vi "finishup.vi"(8 "error in (no error)":errorcluster, 11 "PixelflySettings in":refnum<class "PixelflySettings.lvclass">) -> (0 "error out":errorcluster, 3 "PixelflySettings out":refnum<class "PixelflySettings.lvclass">)   [LabVIEW 2011, in "Tools.lvlib" / "Settings.lvlib" / "PixelflySettings.lvclass"]
uses:
  PixelflySettings.lvclass
  PixelflySettings.lvclass/PixelflySettings.ctl
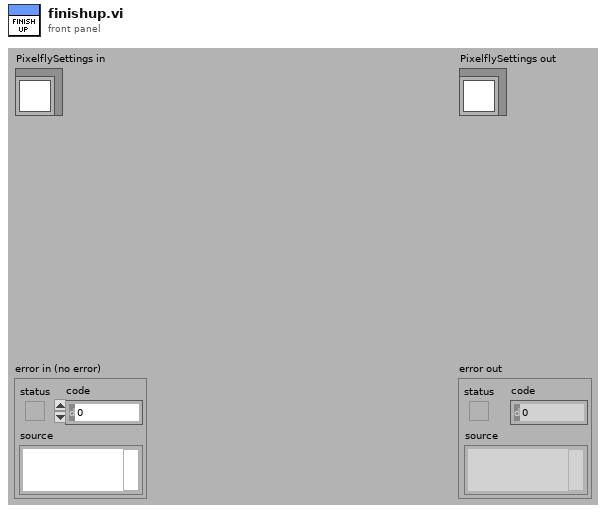
[diagram p1: front panel]
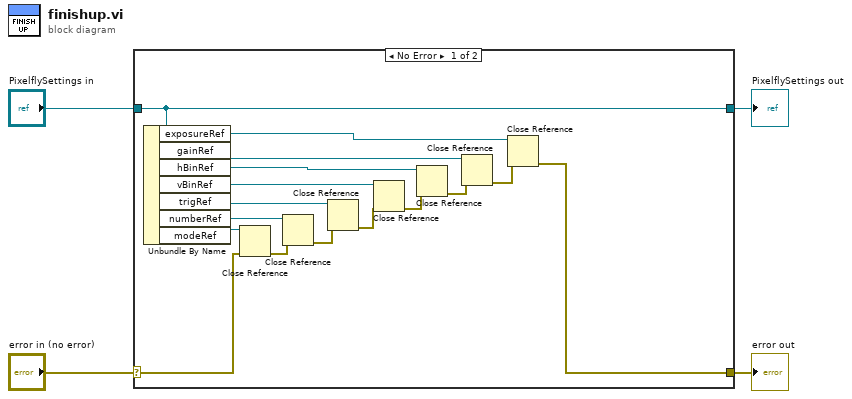
[diagram p0: block diagram]
diagram:
  n1 = case shown="No Error" "error in (no error)" {
    selector: "error in (no error)" -> [w6 w22]
    tunnel: [w5 w22] -> w3
    tunnel: [w20 w21] -> w1
    tunnel: "PixelflySettings in" -> [w20 w21]
    frame No Error {
      n2 = Unbundle By Name(w20) -> ("exposureRef"=w13:refnum<vi>, "gainRef"=w14:refnum<vi>, "hBinRef"=w15:refnum<vi>, "vBinRef"=w16:refnum<vi>, "trigRef"=w17:refnum<vi>, "numberRef"=w18:refnum<vi>, "modeRef"=w19:refnum<vi>)
      n3 = Close Reference(reference=w19, error in (no error)=w6) -> (error out=w12:errorcluster)
      n4 = Close Reference(reference=w18, error in (no error)=w12) -> (error out=w11:errorcluster)
      n5 = Close Reference(reference=w17, error in (no error)=w11) -> (error out=w10:errorcluster)
      n6 = Close Reference(reference=w16, error in (no error)=w10) -> (error out=w9:errorcluster)
      n7 = Close Reference(reference=w15, error in (no error)=w9) -> (error out=w8:errorcluster)
      n8 = Close Reference(reference=w14, error in (no error)=w8) -> (error out=w7:errorcluster)
      n9 = Close Reference(reference=w13, error in (no error)=w7) -> (error out=w5:errorcluster)
    }
    frame Error {
    }
  }
  "error out" <- w3
  "PixelflySettings out" <- w1
